vi "Moisture SASS.vi"() -> (0 "LOW MOISTURE":bool, 1 "INTERMEDIATE MOISTURE":bool, 2 "HIGH MOISTURE":bool, 3 "MOISTURE LEVEL(ppm)":dbl)   [LabVIEW 2013]
uses:
  <vilib>/myRIO/Instrument Drivers/Onboard IO/AI/vis/Smart Open.vi
  <vilib>/myRIO/Instrument Drivers/Onboard IO/AI/vis/Read.vi
  <vilib>/myRIO/Instrument Drivers/Onboard IO/AI/vis/Open.vi
  <vilib>/myRIO/Common/Instrument Driver Framework/myRIO v1.0/AI/vis/myRIO v1.1 Open AI.vi
  <vilib>/myRIO/Common/Instrument Driver Framework/Utilities/vis/Validate Channels.vi
  <vilib>/myRIO/Common/Instrument Driver Framework/myRIO v1.0/AI/vis/myRIO v1.0 Reserve AI.vi
  <vilib>/myRIO/Common/Instrument Driver Framework/myRIO v1.0/AI/vis/myRIO v1.0 Build MUX Configuration AI.vi
  <vilib>/myRIO/Common/Instrument Driver Framework/myRIO v1.0/Resource Manager/vis/myRIO v1.0 Reserve Channel List.vi
  <vilib>/myRIO/Common/Instrument Driver Framework/myRIO v1.0/Resource Manager/vis/myRIO v1.0 Reserve Channel.vi
  <vilib>/myRIO/Common/Instrument Driver Framework/myRIO v1.0/Resource Manager/vis/myRIO v1.0 Unreserve Channel.vi
  <vilib>/myRIO/Common/Instrument Driver Framework/myRIO v1.0/Resource Manager/vis/myRIO v1.0 Build Mutex Name.vi
  <vilib>/myRIO/Common/Instrument Driver Framework/myRIO v1.0/myRIO v1.1 Open.vi
  <vilib>/myRIO/Common/Instrument Driver Framework/myRIO v1.0/AI/vis/myRIO v1.0 Get Scaling Constants AI.vi
  <vilib>/Utility/VariantDataType/GetNumericInfo.vi
  <vilib>/Utility/error.llb/Error Cluster From Error Code.vi
  <vilib>/myRIO/Common/Instrument Driver Framework/Utilities/vis/IO Manager.vi
  <vilib>/myRIO/Common/Instrument Driver Framework/Utilities/vis/Configuration Manager.vi
  <vilib>/myRIO/Common/Instrument Driver Framework/myRIO v1.0/myRIO v1.0 Close.vi
  <vilib>/myRIO/Common/Instrument Driver Framework/myRIO v1.0/AI/vis/myRIO v1.0 Read AI.vi
panel:
  # "AJAY KUMAR GARG ENGINEERING COLLEGE\n                 NI-YANTRA 2017\n                      NIY-135"
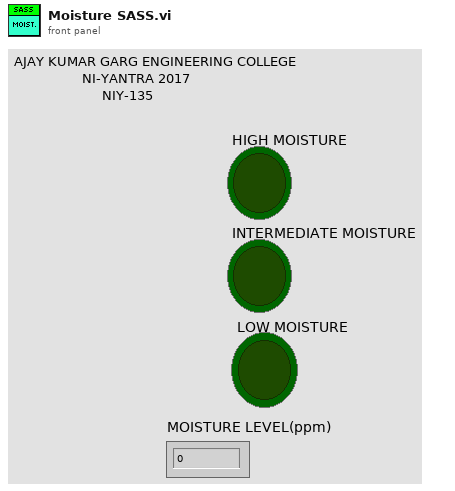
[diagram p1: front panel]
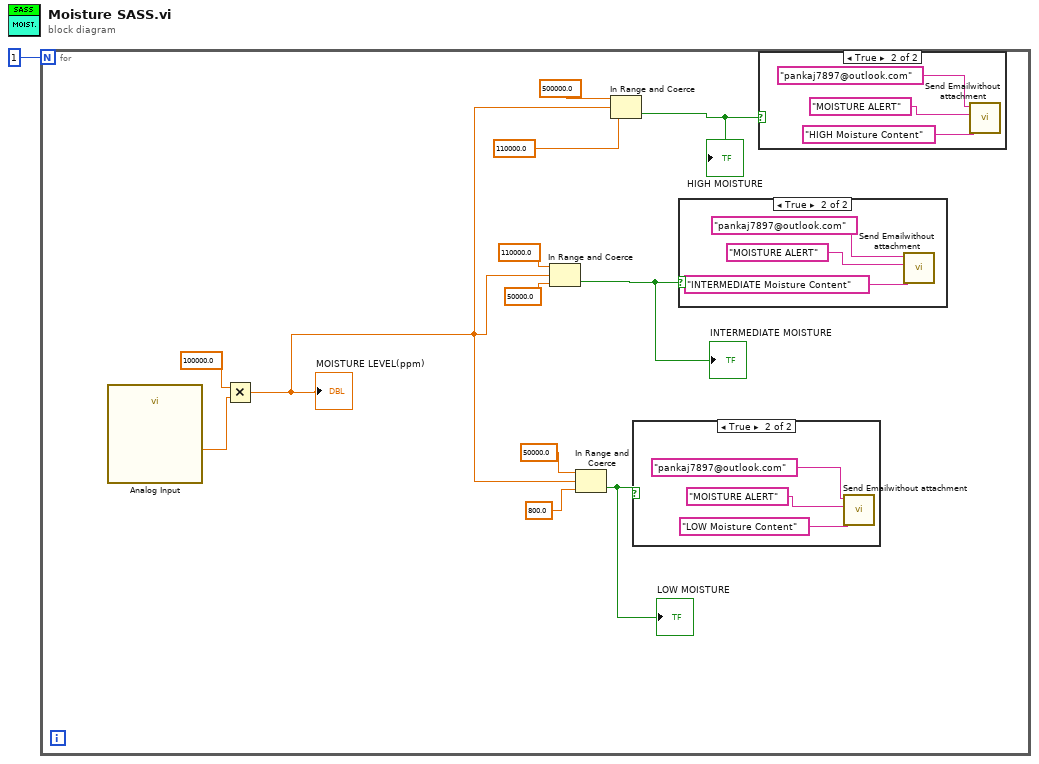
[diagram p0: block diagram]
diagram:
  n1 = for {
    N: 1 -> [_]
    n2 = call "Analog Input"() -> ("A/AI0 (Pin 3)"=w13:dbl)  [unwired: 26 in, 1 out]
    n3 = Multiply(x=100000.0, y=w13) -> (x*y=w4:dbl)
    "MOISTURE LEVEL(ppm)" <- w4
    n4 = In Range and Coerce(upper limit=110000.0, x=w4, lower limit=50000.0 ("upper limit")) -> (In Range?=w3:bool)  [unwired: 1 out]
    "INTERMEDIATE MOISTURE" <- w3
    n5 = In Range and Coerce(upper limit=50000.0, x=w4, lower limit=800.0 ("upper limit")) -> (In Range?=w2:bool)  [unwired: 1 out]
    "LOW MOISTURE" <- w2
    n6 = In Range and Coerce(upper limit=500000.0, x=w4, lower limit=110000.0 ("upper limit")) -> (In Range?=w5:bool)  [unwired: 1 out]
    "HIGH MOISTURE" <- w5
    n7 = case shown="True" w2 {
      frame False {
      }
      frame True {
        n8 = call "Send Emailwithout attachment.vi"("To: 2"="pankaj7897@outlook.com", "Subject 2"="MOISTURE ALERT", "Message 2"="LOW Moisture Content") -> ()  [unwired: 8 in]
      }
    }
    n9 = case shown="True" w3 {
      frame False {
      }
      frame True {
        n10 = call "Send Emailwithout attachment.vi"("To: 2"="pankaj7897@outlook.com", "Subject 2"="MOISTURE ALERT", "Message 2"="INTERMEDIATE Moisture Content") -> ()  [unwired: 8 in]
      }
    }
    n11 = case shown="True" w5 {
      frame False {
      }
      frame True {
        n12 = call "Send Emailwithout attachment.vi"("To: 2"="pankaj7897@outlook.com", "Subject 2"="MOISTURE ALERT", "Message 2"="HIGH Moisture Content") -> ()  [unwired: 8 in]
      }
    }
  }
